vi "Write MessageReceiveQueue.vi"(8 "error in (no error)":errorcluster, 10 "MessageReceiveQueue":refnum<queue>, 11 "MQTT Client in":refnum<class "MQTT Client.lvclass">) -> (0 "error out":errorcluster, 3 "MQTT Client out":refnum<class "MQTT Client.lvclass">)   [LabVIEW 2020, in "MQTT Client.lvclass"]
uses:
  MQTT Client.lvclass
  mqttMessage.ctl
  MQTT Client.lvclass/MQTT Client.ctl
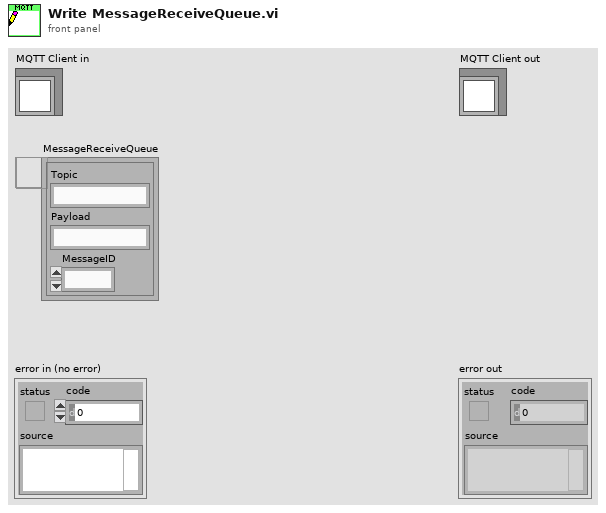
[diagram p1: front panel]
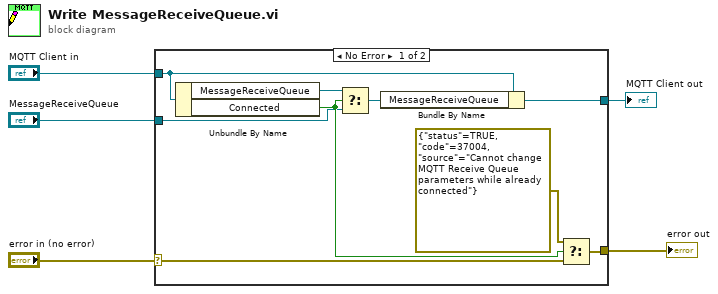
[diagram p0: block diagram]
diagram:
  n1 = case shown="No Error" "error in (no error)" {
    selector: "error in (no error)" -> [w12 w15]
    tunnel: [w11 w15] -> w3
    tunnel: [w14 w16] -> w2
    tunnel: "MQTT Client in" -> [w13 w16]
    tunnel: "MessageReceiveQueue" -> [w7 _]
    frame No Error {
      n2 = Unbundle By Name(w13) -> ("MessageReceiveQueue"=w9:refnum<queue>, "Connected"=w8:bool)
      n3 = Select(t=w9, s=w8, f=w7) -> (s? t:f=w6:refnum<queue>)
      n4 = Bundle By Name(cluster=w13, "MessageReceiveQueue"=w6) -> (w14:refnum<class "MQTT Client.lvclass">)
      n5 = Select(t=errorcluster {"status"=TRUE, "code"=37004, "source"="Cannot change MQTT Receive Queue parameters while already connected"}, s=w8, f=w12) -> (s? t:f=w11:errorcluster)
    }
    frame Error {
    }
  }
  "error out" <- w3
  "MQTT Client out" <- w2
